vi "Read Childs.vi"(8 "error in (no error)":errorcluster, 11 "cClass in":refnum<class "baseClass.lvclass">) -> (0 "error out":errorcluster, 2 "Childs":string[](array[string]), 3 "cClass out":refnum<class "baseClass.lvclass">)   [LabVIEW 2013, in "baseClass.lvclass"]
uses:
  baseClass.lvclass
  baseClass.lvclass/baseClass.ctl
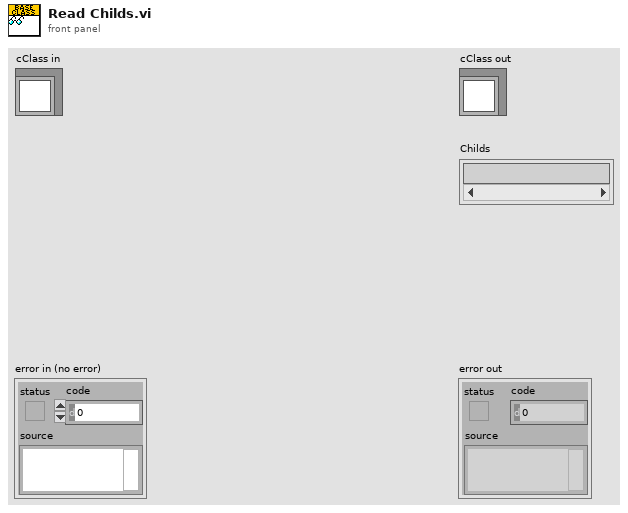
[diagram p1: front panel]
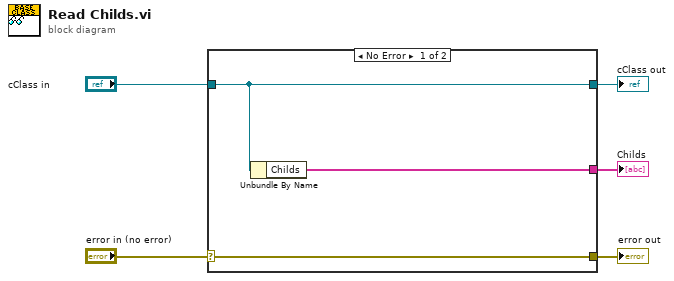
[diagram p0: block diagram]
diagram:
  n1 = case shown="No Error" "error in (no error)" {
    selector: "error in (no error)" -> [w8 w9]
    tunnel: [w8 w9] -> w4
    tunnel: [w7 w10] -> w2
    tunnel: "cClass in" -> [w7 w10]
    tunnel: [w6 _] -> w1
    frame No Error {
      n2 = Unbundle By Name(w7) -> ("Childs"=w6:string[])
    }
    frame Error {
    }
  }
  "error out" <- w4
  "cClass out" <- w2
  "Childs" <- w1
